vi "fgt set all Valves.vi"(8 "error in (no error)":errorcluster, 9 "position":i32, 10 "moduleIndex":u32, 11 "controllerIndex":u32) -> (0 "error out":errorcluster)   [LabVIEW 2016, in "fgt_SDK.lvlib"]
doc: "Sets the position of all two positional valves connected to specified controller / module."
uses:
  fgt_SDK.lvlib
  dlls/fgt_SDK_32.dll
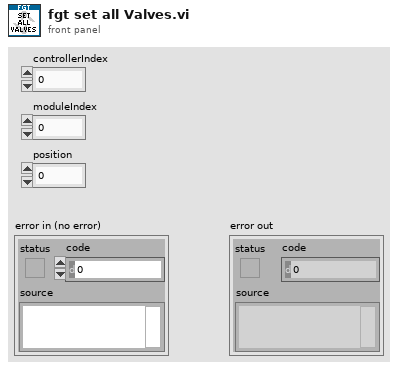
[diagram p1: front panel]
types:
  T1 = typedef "fgt_SDK.lvlib/fgt_STATUS_INFO.ctl" = cluster{"InstrType":T2, "instrSN":u16, "errorCode":u8, "infoCode":u8, "detail":string}
  T2 = typedef "fgt_SDK.lvlib/fgt_INSTRUMENT_TYPE.ctl" = enum32{"None", "MFCS", "MFCS_EZ", "FRP", "LineUP", "IPS", "ESS", "F_OEM"}
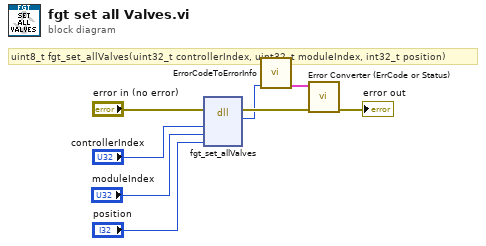
[diagram p0: block diagram]
diagram:
  # "uint8_t fgt_set_allValves(uint32_t controllerIndex, uint32_t moduleIndex, int32_t position)"
  n1 = dll-call lib="C:/projects/SDK/fgt-sdk-labview/dlls/fgt_SDK_*.*" fn="fgt_set_allValves"(error in="error in (no error)", "controllerIndex"="controllerIndex", "moduleIndex"="moduleIndex", "position"="position") -> (error out=w6:errorcluster, "return type"=w4:u8)  [unwired: 5 in, 1 out]
  n2 = call "ErrorCodeToErrorInfo.vi"("return type"=w4) -> ("StatusInfo"=w3:T1)  [unwired: 10 in]
  n3 = call "Error Converter (ErrCode or Status).vi"("error in (no error)"=w6, "StatusInfo"=w3) -> ("error out"=→"error out":errorcluster)  [unwired: 9 in]
